vi "createOutboundChannel.vi"(8 "error in (no error)":errorcluster, 10 "redirect":string, 11 "Connection.NetworkStream in":refnum<class "Connection.NetworkStream.lvclass">) -> (0 "error out":errorcluster, 3 "Connection.NetworkStream out":refnum<class "Connection.NetworkStream.lvclass">)   [LabVIEW 2013, in "Connection.NetworkQueue_GOSPL.lvlib" / "Connection.NetworkStream.lvclass"]
uses:
  Connection.NetworkStream.lvclass
  Connection.NetworkStream.lvclass/Connection.NetworkStream.ctl
  Connection/Connection.lvclass/Connection.ctl
  Connection/Connection.lvclass
  <vilib>/LabVIEW Open Source Project/Unicity/RandomStringGenerator/RandomStringGenerator.lvclass
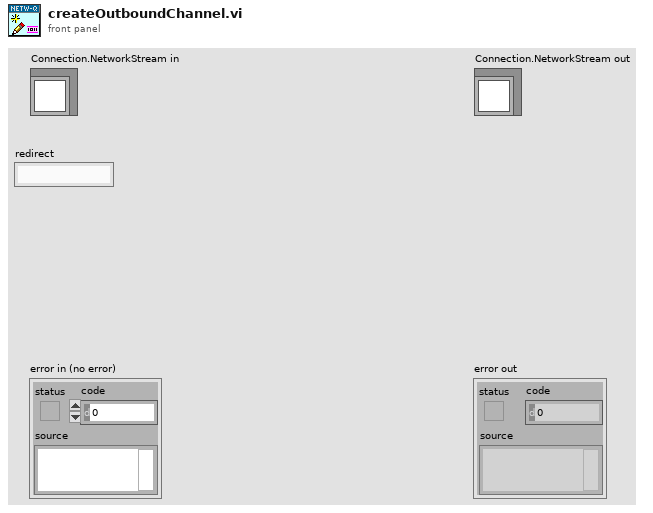
[diagram p1: front panel]
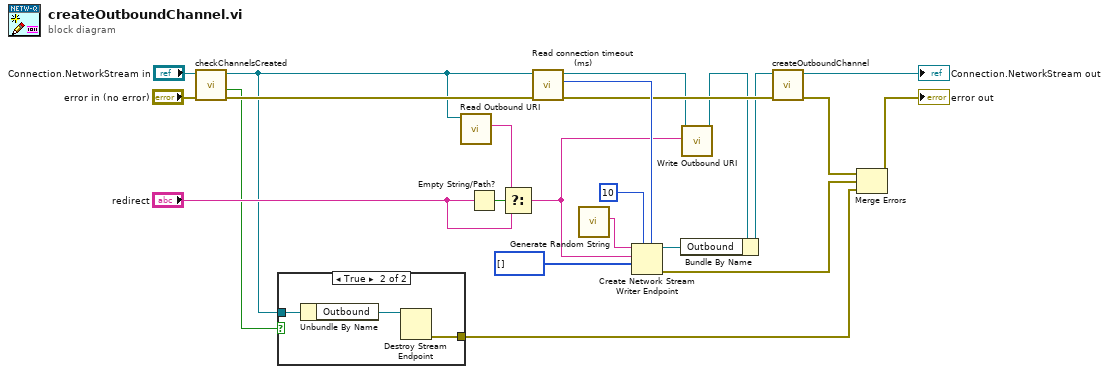
[diagram p0: block diagram]
diagram:
  n1 = call-dynamic "checkChannelsCreated.vi"("error in (no error)"="error in (no error)", "Connection.NetworkStream in"="Connection.NetworkStream in") -> ("error out"=w12:errorcluster, "outbound created"=w1:bool, "Connection.NetworkStream out"=w3:refnum<class "Connection.NetworkStream.lvclass">)  [unwired: 6 in, 1 out]
  n2 = case shown="True" w1 {
    tunnel: w3 -> [_ w26]
    tunnel: [_ w24] -> w2
    frame False {
    }
    frame True {
      n3 = Unbundle By Name(w26) -> ("Outbound"=w25:refnum<k21>)
      n4 = Destroy Stream Endpoint(11:w25) -> (0:w24:errorcluster)  [unwired: 1 in]
    }
  }
  n5 = call "Read Outbound URI.vi"("Connection in"=w3) -> ("Outbound URI"=w7:string)  [unwired: 9 in, 1 out]
  n6 = Empty String/Path?(string/path="redirect") -> (empty?=w14:bool)
  n7 = Select(t=w7, s=w14, f="redirect") -> (s? t:f=w6:string)
  n8 = call "Read connection timeout (ms).vi"("error in (no error)"=w12, "Connection in"=w3) -> ("error out"=w11:errorcluster, "connection timeout (ms)"=w18:i32, "Connection out"=w5:refnum<class "Connection.NetworkStream.lvclass">)  [unwired: 7 in]
  n9 = call <vilib>:"Generate Random String.vi"() -> ("Random String"=w19:string)  [unwired: 11 in]
  n10 = Create Network Stream Writer Endpoint(5:w18, 7:10 ("writer buffer size"), 9:u8[] [] ("Bytes Stream"), 10:w6, 11:w19) -> (0:w15:errorcluster, 3:w10:refnum<k21>)  [unwired: 2 in]
  n11 = call "Write Outbound URI.vi"("Outbound URI"=w6, "Connection in"=w5) -> ("Connection out"=w4:refnum<class "Connection.NetworkStream.lvclass">)  [unwired: 9 in]
  n12 = Bundle By Name(cluster=w4, "Outbound"=w10) -> (w9:refnum<class "Connection.NetworkStream.lvclass">)
  n13 = call-parent "createOutboundChannel.vi"("error in (no error)"=w11, "Connection in"=w9) -> ("error out"=w20:errorcluster, "Connection out"=→"Connection.NetworkStream out":refnum<class "Connection.NetworkStream.lvclass">)  [unwired: 8 in]
  n14 = Merge Errors(w20, w15, w2) -> (→"error out":errorcluster)
